vi "ParseVectorFile.SVG.PathFactory.vi"(8 "error in (no error)":errorcluster, 11 "ParseVectorFile in":refnum<class "ParseVectorFile.lvclass">) -> (0 "error out":errorcluster, 3 "ParseVectorFile out":refnum<class "ParseVectorFile.lvclass">)   [LabVIEW 2019, in "ParseVectorFile.lvclass"]
uses:
  ParseVectorFile.lvclass
  ParseVectorFile.lvclass/ParseVectorFile.ctl
  ParseXML/ParseSVG.lvclass/ParseSVG.ctl
  ParsePaths/Path.lvclass
  ParseXML/ParseSVG.lvclass
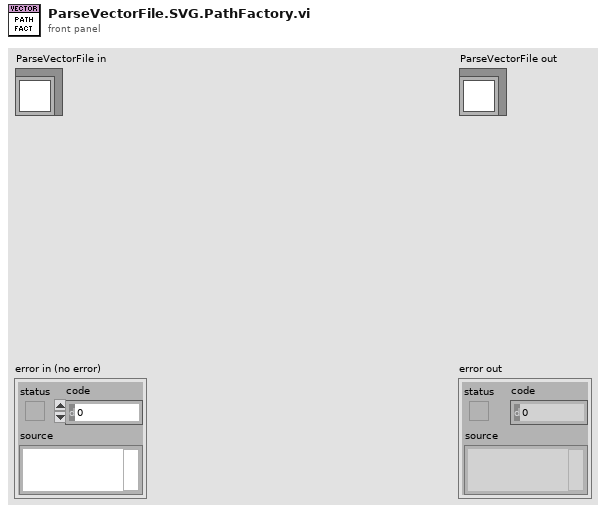
[diagram p1: front panel]
types:
  T1 = typedef "ParseSVG.lvclass/Path.ctl" = cluster{"d":string, "style":string, "transform":string}
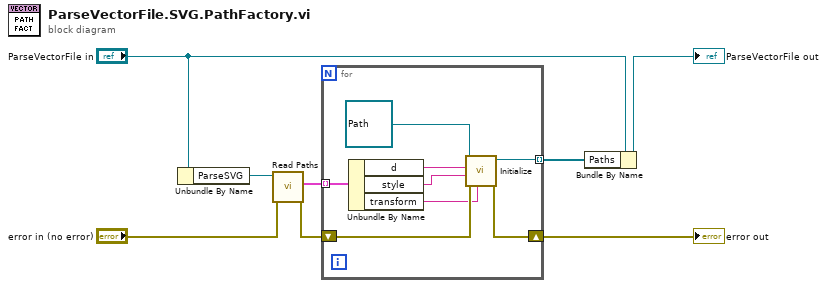
[diagram p0: block diagram]
diagram:
  n1 = Unbundle By Name("ParseVectorFile in") -> ("ParseSVG"=w8:refnum<class "ParseSVG.lvclass">)
  n2 = call "Read Paths.vi"("error in (no error)"="error in (no error)", "ParseXML in"=w8) -> ("error out"=w3:errorcluster, "Paths"=w5:T1[])  [unwired: 7 in, 1 out]
  n3 = for {
    tunnel: w5 -> [w16] mode=indexing
    shift-right: [w11] -> w2
    shift-left: w3 -> [w12]
    tunnel: [w9] -> w1 mode=indexing
    n4 = Unbundle By Name(w16) -> ("d"=w15:string, "style"=w14:string, "transform"=w10:string)
    n5 = call "Initialize.vi"("Path Transform"=w10, "error in (no error)"=w12, "Path Style"=w14, "Path Data"=w15, "Path in"=refnum<class "Path.lvclass"> refnum ("Path.lvclass")) -> ("error out"=w11:errorcluster, "Path out"=w9:refnum<class "Path.lvclass">)  [unwired: 5 in]
  }
  "error out" <- w2
  n6 = Bundle By Name(cluster="ParseVectorFile in", "Paths"=w1) -> (→"ParseVectorFile out":refnum<class "ParseVectorFile.lvclass">)
